vi "Teleop.vi"(0 "Call Context":T9) -> (6 "SubState 3":T4, 9 "SubState 4":T8, 11 "Loop 3 Data":T3, 14 "SubState 0":T4=enum."driver control", 15 "Loop 1 Data":T6, 16 "Loop 0 Data":T7, 17 "SubState 1":T4, 18 "Loop 2 Data":T5, 19 "SubState 2":T4)   [LabVIEW 2013]
uses:
  typedefs/subStates.ctl
  <vilib>/Rock Robotics/WPI/DriverStation/WPI_DriverStationDerivedRobotMode.ctl
  typedefs/singleUseSubstate.ctl
  typedefs/Loop Datatypes/Loop 0 Datatype.ctl
  typedefs/Loop Datatypes/Loop 1 Datatype.ctl
  typedefs/Loop Datatypes/Loop 2 Datatype.ctl
  typedefs/Loop Datatypes/Loop 3 Datatype.ctl
  <vilib>/Rock Robotics/WPI/Joystick/WPI_JoystickDevRef.ctl
  <vilib>/Rock Robotics/WPI/Joystick/WPI_JoystickDeviceEnum.ctl
  typedefs/fg_typedef.ctl
  typedefs/vision enable.ctl
  <vilib>/Rock Robotics/WPI/Joystick/WPI_JoystickGetSetRefNum.vi
panel:
  out "JS3":T1
  out "Drive to DC":bool
  out "JS1":T1
  out "JS2":T1
  out "Exit Value":i32=-1
  # "Loop Data and Substates"
  # "Drive Loop"
  # "State Machine Master Loop"
  # "Pickup/Passing Belts Loop"
  # "Pickup/Passing Arm Loop"
  # "Pneumatics Loop"
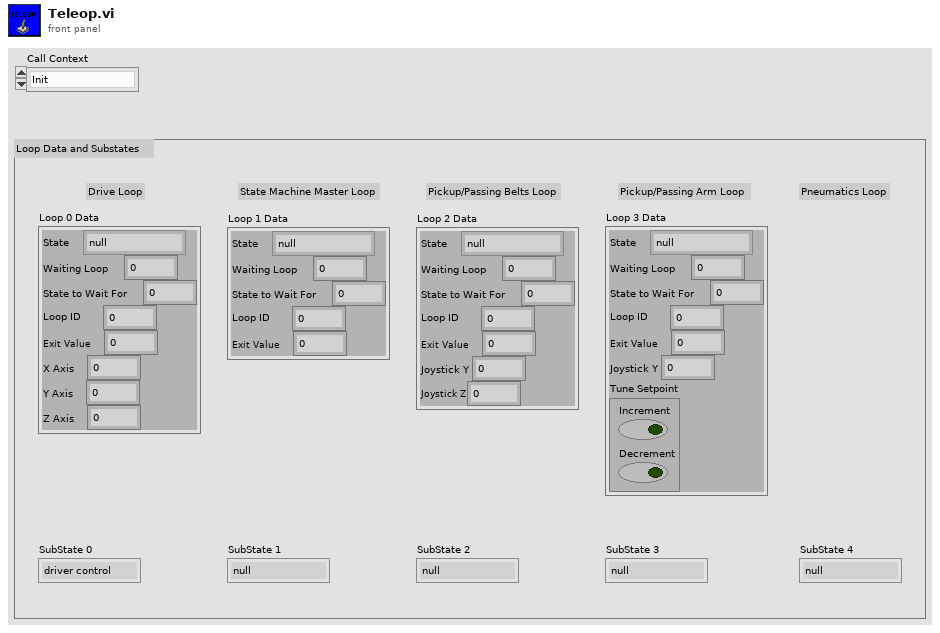
[diagram p1: front panel]
types:
  T1 = typedef "WPI_JoystickDevRef.ctl" = cluster{"Device":T2}
  T2 = typedef "WPI_JoystickDeviceEnum.ctl" = enum16{"USB 1", "USB 2", "USB 3", "USB 4", "Kinect 1", "Kinect 2"}
  T3 = typedef "Loop 3 Datatype.ctl" = cluster{"State":T4, "Waiting Loop":i32, "State to Wait For":i32, "Loop ID":i32, "Exit Value":i32, "Joystick Y":dbl, "Tune Setpoint":cluster{"Increment":bool, "Decrement":bool}}
  T4 = typedef "subStates.ctl" = enum16{"null", "wait", "driver control", "auto", "manual override", "hold position", "rotate", "pickup", "pass", "load", "goto shoot", "shoot high goal", "shoot low goal", "cancel arm", "cancel shooter", "end"}
  T5 = typedef "Loop 2 Datatype.ctl" = cluster{"State":T4, "Waiting Loop":i32, "State to Wait For":i32, "Loop ID":i32, "Exit Value":i32, "Joystick Y":dbl, "Joystick Z":dbl}
  T6 = typedef "Loop 1 Datatype.ctl" = cluster{"State":T4, "Waiting Loop":i32, "State to Wait For":i32, "Loop ID":i32, "Exit Value":i32}
  T7 = typedef "Loop 0 Datatype.ctl" = cluster{"State":T4, "Waiting Loop":i32, "State to Wait For":i32, "Loop ID":i32, "Exit Value":i32, "X Axis":dbl, "Y Axis":dbl, "Z Axis":dbl}
  T8 = typedef "singleUseSubstate.ctl" = enum16{"null", "wait", "shift high", "shift low", "extend shooter", "retract shooter", "latch", "unlatch", "end"}
  T9 = typedef "WPI_DriverStationDerivedRobotMode.ctl" = enum16{"Init", "Execute", "Stop"}
  T10 = cluster{"axis 1 (x)":dbl, "axis 2 (y)":dbl, "axis 3 (throttle)":dbl, "axis 4":dbl, "axis 5":dbl, "axis 6":dbl}
  T11 = typedef "WPI_EncoderDevRef.ctl" = cluster{"DevStatus":errorcluster, "EncoderIndex":T12, "CounterIndex":T13, "DistancePerCount":dbl, "Decoding Type":T14}
  T12 = typedef "FPGA_EncoderIdx.ctl" = enum8{"Enc 0", "Enc 1", "Enc 2", "Enc 3", "Invalid"}
  T13 = typedef "FPGA_CounterCtrSystemIndex.ctl" = enum8{"Ctr 0", "Ctr 1", "Ctr 2", "Ctr 3", "Ctr 4", "Ctr 5", "Ctr 6", "Ctr 7", "Invalid"}
  T14 = typedef "WPI_EncoderType.ctl" = enum16{"1x", "2x", "4x"}
  T15 = typedef "vision enable.ctl" = enum16{"Enable", "Disable", "Stop"}
  T16 = typedef "fg_typedef.ctl" = enum16{"Get", "Set"}
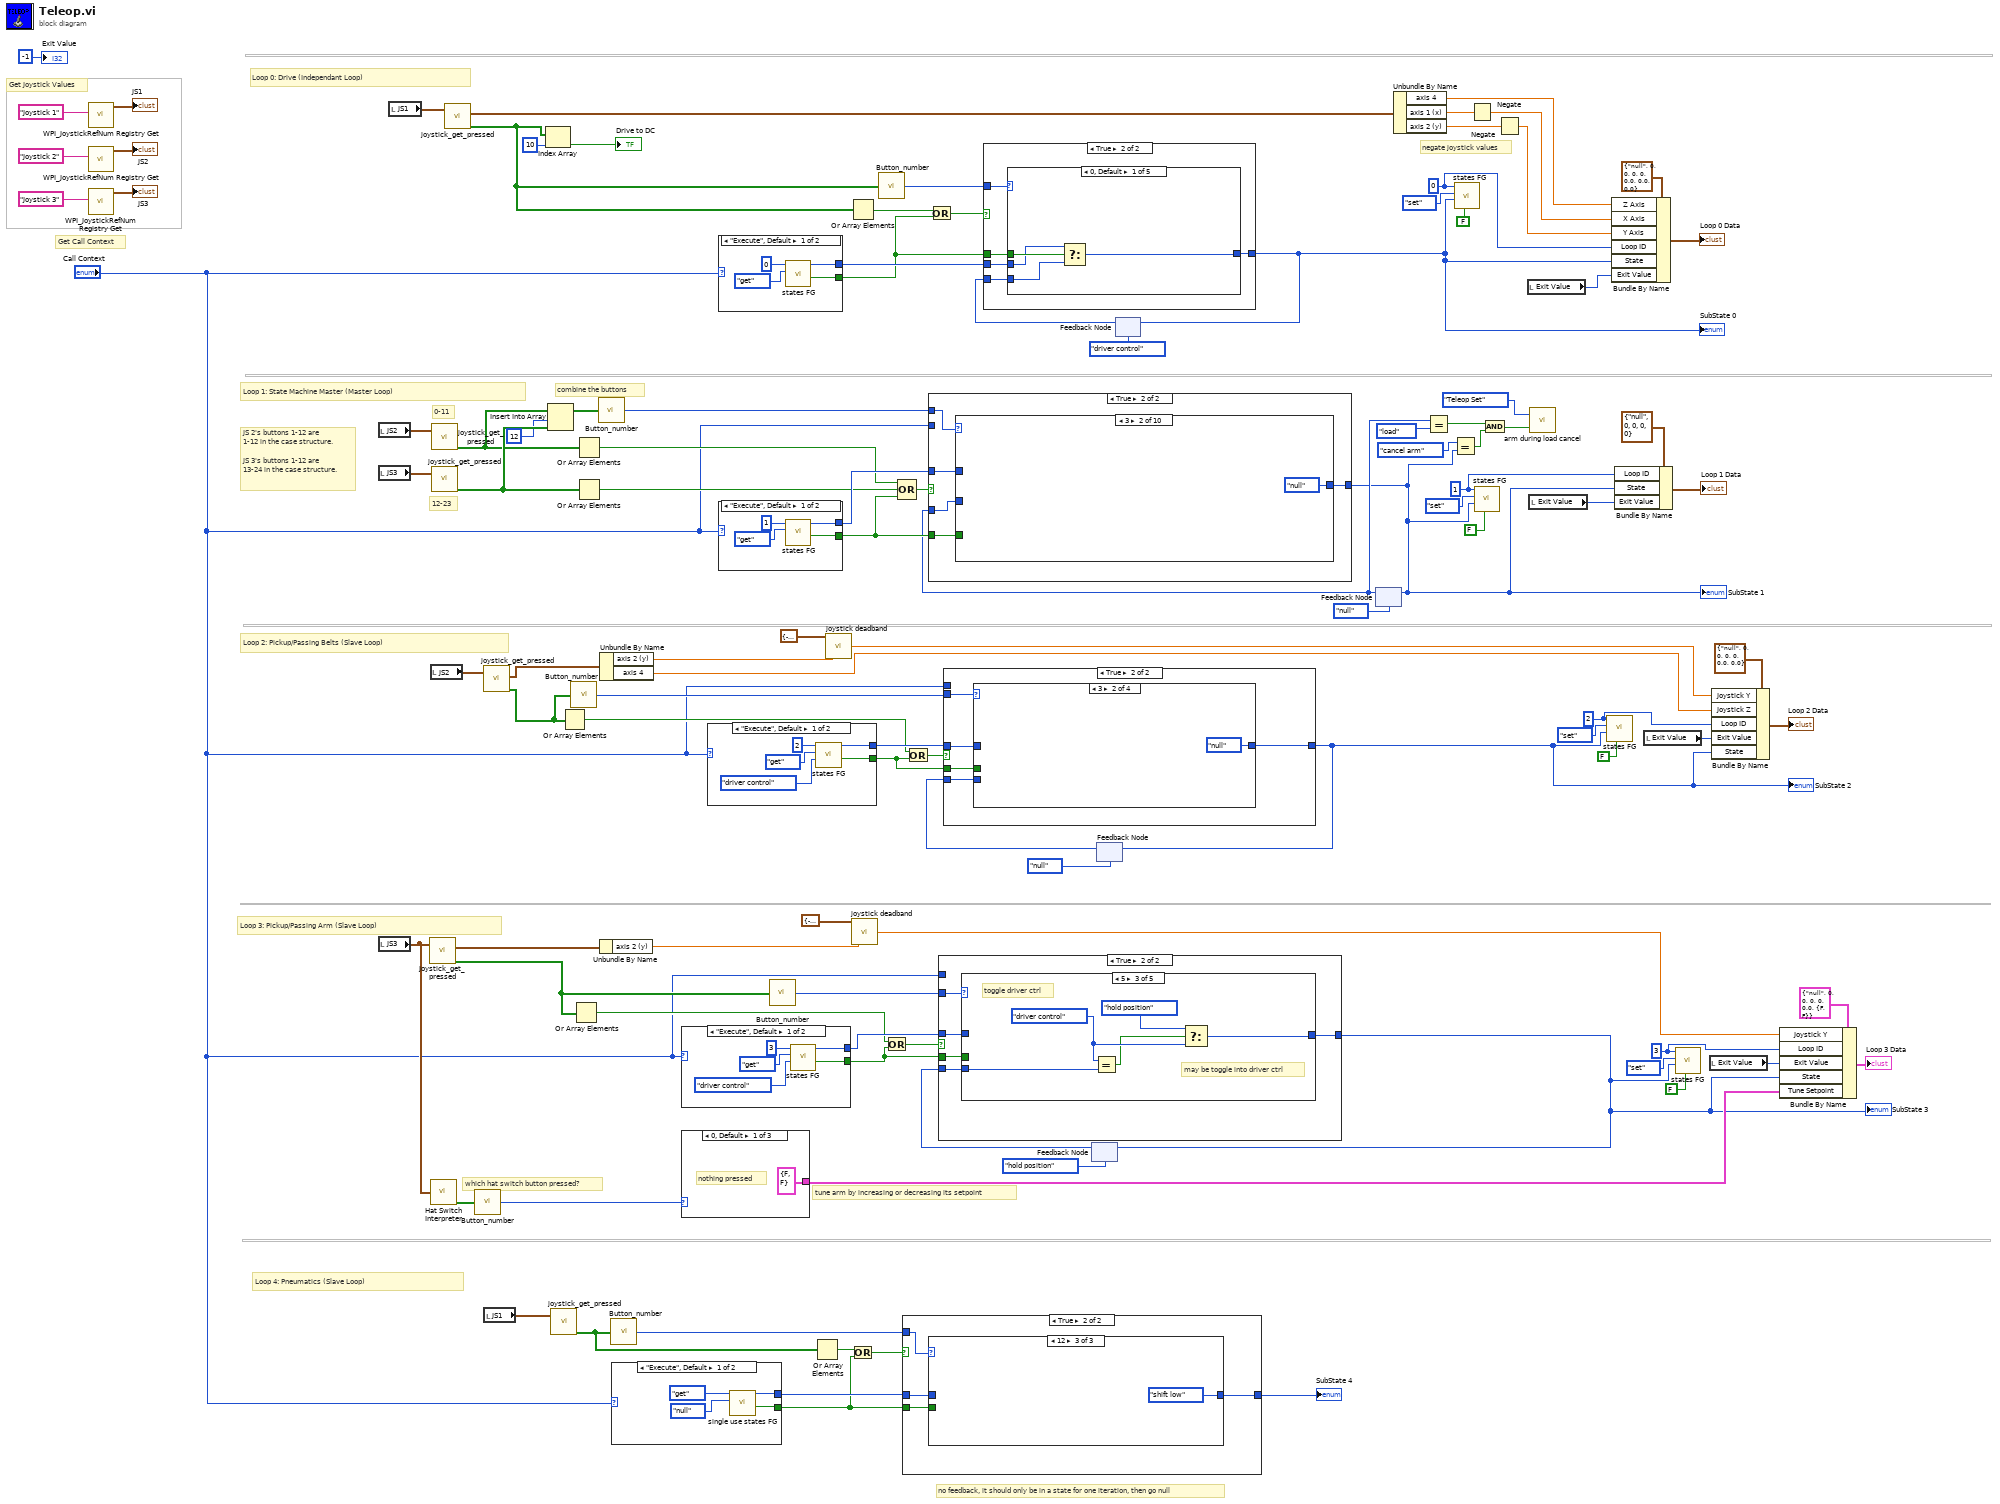
[diagram p0: block diagram]
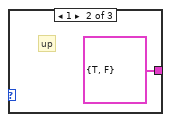
[diagram p2: hidden frame]
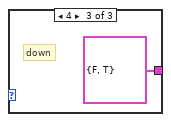
[diagram p3: hidden frame]
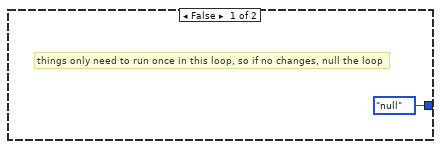
[diagram p4: hidden frame]
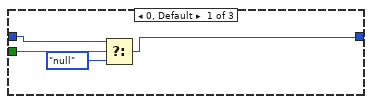
[diagram p5: hidden frame]
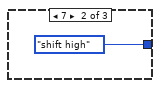
[diagram p6: hidden frame]
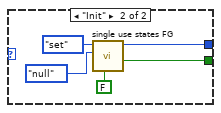
[diagram p7: hidden frame]
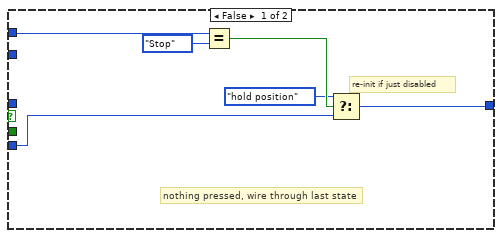
[diagram p8: hidden frame]
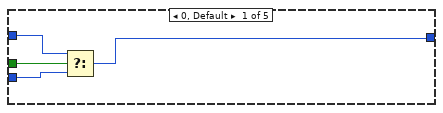
[diagram p9: hidden frame]
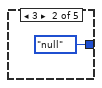
[diagram p10: hidden frame]
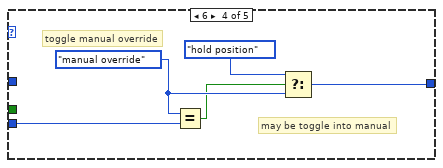
[diagram p11: hidden frame]
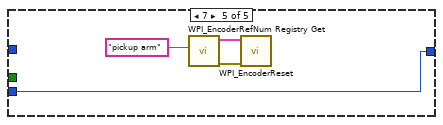
[diagram p12: hidden frame]
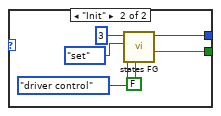
[diagram p13: hidden frame]
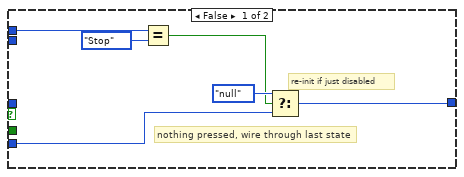
[diagram p14: hidden frame]
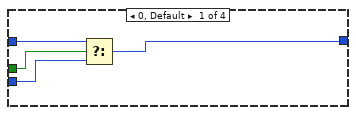
[diagram p15: hidden frame]
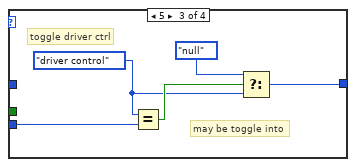
[diagram p16: hidden frame]
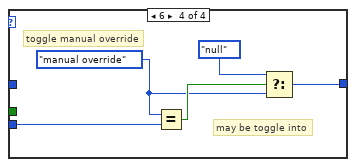
[diagram p17: hidden frame]
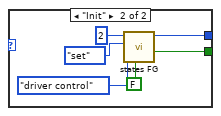
[diagram p18: hidden frame]
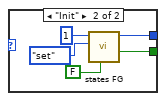
[diagram p19: hidden frame]
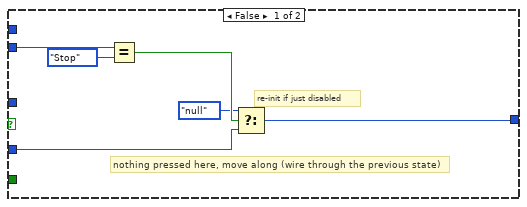
[diagram p20: hidden frame]
diagram:
  w84 = 3 ("Loop ID")
  w85 = 2 ("Loop ID")
  w94 = 1 ("Loop ID")
  w96 = 0 ("Loop ID")
  # "no feedback, it should only be in a state for one iteration, then go null"
  # "JS 2's buttons 1-12 are\n1-12 in the case structure.\n\nJS 3's buttons 1-12 are\n13-24 in the case structure."
  # "combine the buttons"
  # "12-23"
  # "0-11"
  # "tune arm by increasing or decreasing its setpoint"
  # "which hat switch button pressed?"
  # "negate joystick values"
  # "Get Call Context"
  # "Get Joystick Values"
  # "Loop 3: Pickup/Passing Arm (Slave Loop)"
  # "Loop 4: Pneumatics (Slave Loop)"
  # "Loop 2: Pickup/Passing Belts (Slave Loop)"
  # "Loop 1: State Machine Master (Master Loop)"
  # "Loop 0: Drive (Independant Loop)"
  n1 = call <vilib>:"WPI_JoystickRefNum Registry Get.vi"("refnum name"="Joystick 1") -> ("JoystickDevRef"=→"JS1":T1)  [unwired: 9 in, 1 out]
  n2 = call <vilib>:"WPI_JoystickRefNum Registry Get.vi"("refnum name"="Joystick 2") -> ("JoystickDevRef"=→"JS2":T1)  [unwired: 9 in, 1 out]
  n3 = call <vilib>:"WPI_JoystickRefNum Registry Get.vi"("refnum name"="Joystick 3") -> ("JoystickDevRef"=→"JS3":T1)  [unwired: 9 in, 1 out]
  n4 = local read "JS2"() -> (w64:T1)
  n5 = local read "JS3"() -> (w16:T1)
  n6 = local read "JS3"() -> (w29:T1)
  n7 = local read "JS1"() -> (w65:T1)
  n8 = call "joystick_get_pressed.vi"("JoystickDevRef 2"=w29) -> ("Axes"=w54:T10, "Buttons Pressed?"=w36:bool[])  [unwired: 1 in, 2 out]
  n9 = local read "JS2"() -> (w42:T1)
  n10 = call "Hat Switch Interpreter.vi"("JoystickDevRef"=w29) -> ("Buttons"=w28:bool[])  [unwired: 4 out]
  n11 = call "joystick_get_pressed.vi"("JoystickDevRef 2"=w64) -> ("Buttons Pressed?"=w12:bool[])  [unwired: 1 in, 3 out]
  n12 = call "joystick_get_pressed.vi"("JoystickDevRef 2"=w16) -> ("Buttons Pressed?"=w13:bool[])  [unwired: 1 in, 3 out]
  n13 = call "joystick_get_pressed.vi"("JoystickDevRef 2"=w65) -> ("Axes"=w69:T10, "Buttons Pressed?"=w47:bool[])  [unwired: 1 in, 2 out]
  n14 = call "Button_number.vi"("Button Array"=w28) -> ("Button Pressed"=w27:i32)
  n15 = call "joystick_get_pressed.vi"("JoystickDevRef 2"=w42) -> ("Axes"=w32:T10, "Buttons Pressed?"=w33:bool[])  [unwired: 1 in, 2 out]
  n16 = local read "JS1"() -> (w45:T1)
  n17 = Index Array(array=w47, index=10) -> (element=→"Drive to DC":bool)
  n18 = Insert Into Array(array=w12, index=12, new element=w13) -> (w10:bool[])
  n19 = call "joystick_get_pressed.vi"("JoystickDevRef 2"=w45) -> ("Buttons Pressed?"=w20:bool[])  [unwired: 1 in, 3 out]
  n20 = Or Array Elements(Boolean array=w33) -> (logical OR=w41:bool)
  n21 = call "Button_number.vi"("Button Array"=w33) -> ("Button Pressed"=w40:i32)
  n22 = Or Array Elements(Boolean array=w36) -> (logical OR=w53:bool)
  n23 = Or Array Elements(Boolean array=w12) -> (logical OR=w15:bool)
  n24 = Or Array Elements(Boolean array=w13) -> (logical OR=w14:bool)
  n25 = call "Button_number.vi"("Button Array"=w10) -> ("Button Pressed"=w58:i32)
  n26 = Unbundle By Name(w54) -> ("axis 2 (y)"=w50:dbl)
  n27 = Unbundle By Name(w32) -> ("axis 2 (y)"=w35:dbl, "axis 4"=w30:dbl)
  n28 = call "Button_number.vi"("Button Array"=w20) -> ("Button Pressed"=w19:i32)
  n29 = case shown="\"Execute\", Default" "Call Context" {
    tunnel: [w114 w117] -> w18
    tunnel: [w115 w116] -> w34
    frame "Execute", Default {
      n30 = call "single use states FG.vi"("substate"=singleUseSubstate."null" ("Enum"), "menu (get)"=enum16{"set", "get"}."get") -> ("exit out"=w114:bool, "substate out"=w115:T8)  [unwired: 6 in, 2 out]
    }
    frame "Init" {
      n31 = call "single use states FG.vi"("exit in"=FALSE, "substate"=singleUseSubstate."null", "menu (get)"=enum16{"set", "get"}."set") -> ("exit out"=w117:bool, "substate out"=w116:T8)  [unwired: 5 in, 2 out]
    }
  }
  n32 = case shown="\"Execute\", Default" "Call Context" {
    tunnel: [w123 w129] -> w51
    tunnel: [w121 w126] -> w82
    frame "Execute", Default {
      n33 = call "states FG.vi"("subState in"=subStates."driver control", "menu (get)"=enum16{"set", "get"}."get", "Loop ID"=3) -> ("exit out"=w123:bool, "subState out"=w121:T4)  [unwired: 5 in, 2 out]
    }
    frame "Init" {
      n34 = call "states FG.vi"("exit in"=FALSE, "subState in"=subStates."driver control", "menu (get)"=enum16{"set", "get"}."set", "Loop ID"=3) -> ("exit out"=w129:bool, "subState out"=w126:T4)  [unwired: 4 in, 2 out]
    }
  }
  n35 = case shown="0, Default" w27 {
    tunnel: [cluster{"Increment":bool, "Decrement":bool} {"Increment"=FALSE, "Decrement"=FALSE} cluster{"Increment":bool, "Decrement":bool} {"Increment"=TRUE, "Decrement"=FALSE} cluster{"Increment":bool, "Decrement":bool} {"Increment"=FALSE, "Decrement"=TRUE}] -> w25
    frame 0, Default {
      # "nothing pressed"
    }
    frame 1 {
      # "up"
    }
    frame 4 {
      # "down"
    }
  }
  n36 = case shown="\"Execute\", Default" "Call Context" {
    tunnel: [w137 w143] -> w56
    tunnel: [w135 w140] -> w100
    frame "Execute", Default {
      n37 = call "states FG.vi"("subState in"=subStates."driver control", "menu (get)"=enum16{"set", "get"}."get", "Loop ID"=2) -> ("exit out"=w137:bool, "subState out"=w135:T4)  [unwired: 5 in, 2 out]
    }
    frame "Init" {
      n38 = call "states FG.vi"("exit in"=FALSE, "subState in"=subStates."driver control", "menu (get)"=enum16{"set", "get"}."set", "Loop ID"=2) -> ("exit out"=w143:bool, "subState out"=w140:T4)  [unwired: 4 in, 2 out]
    }
  }
  n39 = case shown="\"Execute\", Default" "Call Context" {
    tunnel: [w147 w152] -> w62
    tunnel: [w146 w150] -> w99
    frame "Execute", Default {
      n40 = call "states FG.vi"("menu (get)"=enum16{"set", "get"}."get", "Loop ID"=0) -> ("exit out"=w147:bool, "subState out"=w146:T4)  [unwired: 6 in, 2 out]
    }
    frame "Init" {
      n41 = call "states FG.vi"("exit in"=FALSE, "menu (get)"=enum16{"set", "get"}."set", "Loop ID"=0) -> ("exit out"=w152:bool, "subState out"=w150:T4)  [unwired: 5 in, 2 out]
    }
  }
  n42 = case shown="\"Execute\", Default" "Call Context" {
    tunnel: [w156 w161] -> w59
    tunnel: [w155 w159] -> w98
    frame "Execute", Default {
      n43 = call "states FG.vi"("menu (get)"=enum16{"set", "get"}."get", "Loop ID"=1) -> ("exit out"=w156:bool, "subState out"=w155:T4)  [unwired: 6 in, 2 out]
    }
    frame "Init" {
      n44 = call "states FG.vi"("exit in"=FALSE, "menu (get)"=enum16{"set", "get"}."set", "Loop ID"=1) -> ("exit out"=w161:bool, "subState out"=w159:T4)  [unwired: 5 in, 2 out]
    }
  }
  n45 = call "Button_number.vi"("Button Array"=w36) -> ("Button Pressed"=w52:i32)
  n46 = Or Array Elements(Boolean array=w20) -> (logical OR=w21:bool)
  n47 = call "joystick deadband.vi"("Joystick In"=w35, "Deadband Range"=cluster{"Deadband Min":dbl, "Deadband Max":dbl} {"Deadband Min"=-0.05, "Deadband Max"=0.05}) -> ("Joystick Out"=w31:dbl)  [unwired: 4 in]
  n48 = Or Array Elements(Boolean array=w47) -> (logical OR=w63:bool)
  n49 = Or(x=w21, y=w18) -> (x .or. y?=w22:bool)
  n50 = call "joystick deadband.vi"("Joystick In"=w50, "Deadband Range"=cluster{"Deadband Min":dbl, "Deadband Max":dbl} {"Deadband Min"=-0.05, "Deadband Max"=0.05}) -> ("Joystick Out"=w26:dbl)  [unwired: 4 in]
  n51 = call "Button_number.vi"("Button Array"=w47) -> ("Button Pressed"=w68:i32)
  n52 = Or(x=w53, y=w51) -> (x .or. y?=w55:bool)
  n53 = Compound Arithmetic op=OR(w15, w14, w59) -> (w60:bool)
  n54 = case shown="True" w22 {
    tunnel: [singleUseSubstate."null" ("Enum") w165] -> w17
    tunnel: w34 -> [_ w166]
    tunnel: w19 -> [_ w167]
    tunnel: w18 -> [_ w168]
    frame False {
      # "things only need to run once in this loop, so if no changes, null the loop"
    }
    frame True {
      n55 = case shown="12" w167 {
        tunnel: w168 -> [w172 _ _]
        tunnel: w166 -> [w171 _ _]
        tunnel: [w170 singleUseSubstate."shift high" ("Enum") singleUseSubstate."shift low" ("Enum")] -> w165
        frame 0, Default {
          n56 = Select(t=w171, s=w172, f=singleUseSubstate."null") -> (s? t:f=w170:T8)
        }
        frame 7 {
        }
        frame 12 {
        }
      }
    }
  }
  "SubState 4" <- w17
  n57 = Or(x=w41, y=w56) -> (x .or. y?=w57:bool)
  n58 = Or(x=w63, y=w62) -> (x .or. y?=w61:bool)
  n59 = feedback #1(subStates."hold position" ("Drive SubState")) -> (w79:T4)
  n60 = case shown="True" w55 {
    tunnel: w79 -> [w177 w181]
    tunnel: [w176 w182] -> w24
    tunnel: w82 -> [_ w183]
    tunnel: w52 -> [_ w185]
    tunnel: w51 -> [_ w184]
    tunnel: "Call Context" -> [w175 _]
    frame False {
      # "nothing pressed, wire through last state"
      # "re-init if just disabled"
      n61 = Equal?(x=w175, y=WPI_DriverStationDerivedRobotMode."Stop") -> (x = y?=w179:bool)
      n62 = Select(t=subStates."hold position", s=w179, f=w177) -> (s? t:f=w176:T4)
    }
    frame True {
      n63 = case shown="5" w185 {
        tunnel: w184 -> [w189 _ _ _ _]
        tunnel: w181 -> [w188 _ w191 w196 w204]
        tunnel: w183 -> [w187 _ _ _ _]
        tunnel: [w186 subStates."null" ("Drive SubState") w192 w197 w204] -> w182
        frame 0, Default {
          n64 = Select(t=w187, s=w189, f=w188) -> (s? t:f=w186:T4)
        }
        frame 3 {
        }
        frame 5 {
          w194 = subStates."driver control" ("Drive SubState")
          # "may be toggle into driver ctrl"
          # "toggle driver ctrl"
          n65 = Equal?(x=w194, y=w191) -> (x = y?=w193:bool)
          n66 = Select(t=subStates."hold position", s=w193, f=w194) -> (s? t:f=w192:T4)
        }
        frame 6 {
          w200 = subStates."manual override" ("Drive SubState")
          # "may be toggle into manual"
          # "toggle manual override"
          n67 = Equal?(x=w200, y=w196) -> (x = y?=w198:bool)
          n68 = Select(t=subStates."hold position", s=w198, f=w200) -> (s? t:f=w197:T4)
        }
        frame 7 {
          n69 = call <vilib>:"WPI_EncoderRefNum Registry Get.vi"("refnum name"="pickup arm") -> ("error out"=w202:errorcluster, "EncoderDevRef"=w201:T11)  [unwired: 9 in]
          n70 = call <vilib>:"WPI_EncoderReset.vi"("error in (no error)"=w202, "EncoderDevRef"=w201) -> ()  [unwired: 8 in, 2 out]
        }
      }
    }
  }
  "SubState 3" <- w24
  n71 = feedback-in #1(w24) -> ()
  n72 = feedback #2(subStates."null" ("Drive SubState")) -> (w103:T4)
  n73 = case shown="True" w57 {
    tunnel: w103 -> [w206 w212]
    tunnel: [w205 w211] -> w23
    tunnel: w100 -> [_ w213]
    tunnel: w40 -> [_ w215]
    tunnel: w56 -> [_ w214]
    tunnel: "Call Context" -> [w207 _]
    frame False {
      # "re-init if just disabled"
      # "nothing pressed, wire through last state"
      n74 = Equal?(x=w207, y=WPI_DriverStationDerivedRobotMode."Stop") -> (x = y?=w209:bool)
      n75 = Select(t=subStates."null", s=w209, f=w206) -> (s? t:f=w205:T4)
    }
    frame True {
      n76 = case shown="3" w215 {
        tunnel: w214 -> [w219 _ _ _]
        tunnel: w213 -> [w218 _ _ _]
        tunnel: w212 -> [w217 _ w225 w227]
        tunnel: [w216 subStates."null" ("Drive SubState") w221 w226] -> w211
        frame 0, Default {
          n77 = Select(t=w218, s=w219, f=w217) -> (s? t:f=w216:T4)
        }
        frame 3 {
        }
        frame 5 {
          w223 = subStates."driver control" ("Drive SubState")
          # "may be toggle into"
          # "toggle driver ctrl"
          n78 = Equal?(x=w223, y=w225) -> (x = y?=w224:bool)
          n79 = Select(t=subStates."null", s=w224, f=w223) -> (s? t:f=w221:T4)
        }
        frame 6 {
          w228 = subStates."manual override" ("Drive SubState")
          # "may be toggle into"
          # "toggle manual override"
          n80 = Equal?(x=w228, y=w227) -> (x = y?=w230:bool)
          n81 = Select(t=subStates."null", s=w230, f=w228) -> (s? t:f=w226:T4)
        }
      }
    }
  }
  "SubState 2" <- w23
  n82 = feedback-in #2(w23) -> ()
  n83 = feedback #3(subStates."driver control" ("Drive SubState")) -> (w105:T4)
  n84 = case shown="True" w61 {
    tunnel: w105 -> [w231 w233]
    tunnel: [w231 w232] -> w44
    tunnel: w99 -> [_ w234]
    tunnel: w68 -> [_ w236]
    tunnel: w62 -> [_ w235]
    frame False {
      # "keep current state, no change necessary"
    }
    frame True {
      n85 = case shown="0, Default" w236 {
        tunnel: w235 -> [w240 _ _ _ _]
        tunnel: w234 -> [w239 _ _ _ _]
        tunnel: w233 -> [w238 w245 w253 _ _]
        tunnel: [w237 w241 w253 subStates."goto shoot" ("Drive SubState") subStates."driver control" ("Drive SubState")] -> w232
        frame 0, Default {
          n86 = Select(t=w239, s=w240, f=w238) -> (s? t:f=w237:T4)
        }
        frame 1 {
          w242 = subStates."hold position" ("x")
          # "button 1, hold position toggle"
          n87 = Equal?(x=w242, y=w245) -> (x = y?=w244:bool)
          n88 = Select(t=subStates."driver control" ("Drive SubState"), s=w244, f=w242) -> (s? t:f=w241:T4)
        }
        frame 8 {
          w248 = vision_enable."Enable" ("y")
          # "toggle vision"
          n89 = call "vision_fg.vi"("Menu"=fg_typedef."Get") -> ("State Out"=w250:T15)  [unwired: 2 in, 1 out]
          n90 = Equal?(x=w250, y=w248) -> (x = y?=w249:bool)
          n91 = Select(t=vision_enable."Disable" ("y"), s=w249, f=w248) -> (s? t:f=w246:T15)
          n92 = call "vision_fg.vi"("Action"=w246, "Menu"=fg_typedef."Set") -> ()  [unwired: 1 in, 2 out]
        }
        frame 10 {
          # "go to shoot location"
          n93 = call "vision_fg.vi"("Action"=vision_enable."Enable", "Menu"=fg_typedef."Set") -> ()  [unwired: 1 in, 2 out]
        }
        frame 11 {
          # "put robot drive in driver control"
          n94 = call "vision_fg.vi"("Action"=vision_enable."Disable", "Menu"=fg_typedef."Set") -> ()  [unwired: 1 in, 2 out]
        }
      }
    }
  }
  "SubState 0" <- w44
  n95 = feedback-in #3(w44) -> ()
  n96 = feedback #4(subStates."null" ("Drive SubState")) -> (w7:T4)
  n97 = case shown="True" w60 {
    tunnel: w7 -> [w262 w269]
    tunnel: [w260 w268] -> w4
    tunnel: w98 -> [_ w270]
    tunnel: w58 -> [_ w267]
    tunnel: w59 -> [_ w266]
    tunnel: "Call Context" -> [w265 _]
    frame False {
      # "re-init if just disabled"
      # "nothing pressed here, move along (wire through the previous state)"
      n98 = Equal?(x=w265, y=WPI_DriverStationDerivedRobotMode."Stop") -> (x = y?=w263:bool)
      n99 = Select(t=subStates."null", s=w263, f=w262) -> (s? t:f=w260:T4)
    }
    frame True {
      n100 = case shown="3" w267 {
        tunnel: w270 -> [w274 _ _ _ _ _ _ _ _ _]
        tunnel: w269 -> [w273 _ _ _ _ _ _ _ _ _]
        tunnel: [w272 subStates."null" ("Drive SubState") subStates."cancel arm" ("Drive SubState") subStates."pickup" ("Drive SubState") subStates."pass" ("Drive SubState") subStates."shoot high goal" ("Drive SubState") subStates."load" ("Drive SubState") subStates."manual override" ("Drive SubState") subStates."shoot low goal" ("Drive SubState") subStates."cancel shooter" ("Drive SubState")] -> w268
        tunnel: w266 -> [w271 _ _ _ _ _ _ _ _ _]
        frame 0, Default {
          n101 = Select(t=w274, s=w271, f=w273) -> (s? t:f=w272:T4)
        }
        frame 3 {
        }
        frame 9 {
          # "button 9, JS 2"
        }
        frame 11 {
          # "button 11, JS 2"
        }
        frame 12 {
          # "button 12, JS 2"
        }
        frame 13 {
          # "button 1, JS 3"
        }
        frame 14 {
          # "button 2, JS 3"
        }
        frame 20 {
          # "manual shoot"
          # "button 8, JS 3"
        }
        frame 23 {
          # "button 11, JS 3"
        }
        frame 24 {
          # "button 12, JS 3"
        }
      }
    }
  }
  "SubState 1" <- w4
  n102 = feedback-in #4(w4) -> ()
  n103 = Unbundle By Name(w69) -> ("axis 4"=w48:dbl, "axis 1 (x)"=w73:dbl, "axis 2 (y)"=w72:dbl)
  n104 = Equal?(x=w7, y=subStates."load") -> (x = y?=w5:bool)
  n105 = Equal?(x=subStates."cancel arm" ("y"), y=w4) -> (x = y?=w6:bool)
  n106 = call "states FG.vi"("exit in"=FALSE, "subState in"=w44, "menu (get)"=enum16{"set", "get"}."set", "Loop ID"=w96) -> ()  [unwired: 4 in, 4 out]
  n107 = Negate(x=w73) -> (-x=w71:dbl)
  n108 = call "states FG.vi"("exit in"=FALSE, "subState in"=w4, "menu (get)"=enum16{"set", "get"}."set", "Loop ID"=w94) -> ()  [unwired: 4 in, 4 out]
  n109 = And(x=w5, y=w6) -> (x .and. y?=w3:bool)
  n110 = Negate(x=w72) -> (-x=w70:dbl)
  n111 = local read "Exit Value"() -> (w92:i32)
  n112 = local read "Exit Value"() -> (w91:i32)
  n113 = call "arm during load cancel.vi"("Arm Canceled During Load?"=w3, "Mode"=enum16{"Get", "Set", "Teleop Set"}."Teleop Set") -> ()  [unwired: 1 out]
  n114 = call "states FG.vi"("exit in"=FALSE, "subState in"=w23, "menu (get)"=enum16{"set", "get"}."set", "Loop ID"=w85) -> ()  [unwired: 4 in, 4 out]
  n115 = Bundle By Name(cluster=T7 {"State"=enum."null", "Waiting Loop"=0, "State to Wait For"=0, "Loop ID"=0, "Exit Value"=0, "X Axis"=0.0, "Y Axis"=0.0, "Z Axis"=0.0} ("Cluster"), "Z Axis"=w48, "X Axis"=w71, "Y Axis"=w70, "Loop ID"=w96, "State"=w44, "Exit Value"=w92) -> (→"Loop 0 Data":T7)
  n116 = Bundle By Name(cluster=T6 {"State"=enum."null", "Waiting Loop"=0, "State to Wait For"=0, "Loop ID"=0, "Exit Value"=0} ("Cluster"), "Loop ID"=w94, "State"=w4, "Exit Value"=w91) -> (→"Loop 1 Data":T6)
  n117 = local read "Exit Value"() -> (w86:i32)
  n118 = call "states FG.vi"("exit in"=FALSE, "subState in"=w24, "menu (get)"=enum16{"set", "get"}."set", "Loop ID"=w84) -> ()  [unwired: 4 in, 4 out]
  n119 = local read "Exit Value"() -> (w83:i32)
  n120 = Bundle By Name(cluster=T5 {"State"=enum."null", "Waiting Loop"=0, "State to Wait For"=0, "Loop ID"=0, "Exit Value"=0, "Joystick Y"=0.0, "Joystick Z"=0.0} ("Loop 2 Data"), "Joystick Y"=w31, "Joystick Z"=w30, "Loop ID"=w85, "Exit Value"=w86, "State"=w23) -> (→"Loop 2 Data":T5)
  n121 = Bundle By Name(cluster=T3 {"State"=enum."null", "Waiting Loop"=0, "State to Wait For"=0, "Loop ID"=0, "Exit Value"=0, "Joystick Y"=0.0, "Tune Setpoint"={"Increment"=FALSE, "Decrement"=FALSE}} ("Loop 3 Data"), "Joystick Y"=w26, "Loop ID"=w84, "Exit Value"=w83, "State"=w24, "Tune Setpoint"=w25) -> (→"Loop 3 Data":T3)
  "Exit Value" <- -1 ("Exit Value")
